vi "Lockin - Format Results.vi"(8 "error in (no error)":errorcluster, 10 "signal in":waveform(dbl)[](array[waveform]), 11 "LockinDAQ":refnum<class "LockinDAQ.lvclass">) -> (0 "error out":errorcluster, 1 "SweepResults":T1, 2 "Results (X,Y,R,Theta)":dbl[][](array[numeric]), 3 "LockinDAQ out":refnum<class "LockinDAQ.lvclass">)   [LabVIEW 2016, in "LockinDAQ.lvclass"]
uses:
  LockinDAQ.lvclass
  Typedefs/SweepResults--Cluster.ctl
  <vilib>/measure/maresamp.llb/Resample Waveform (single shot).vi
  <vilib>/measure/NI_MAPro.lvlib
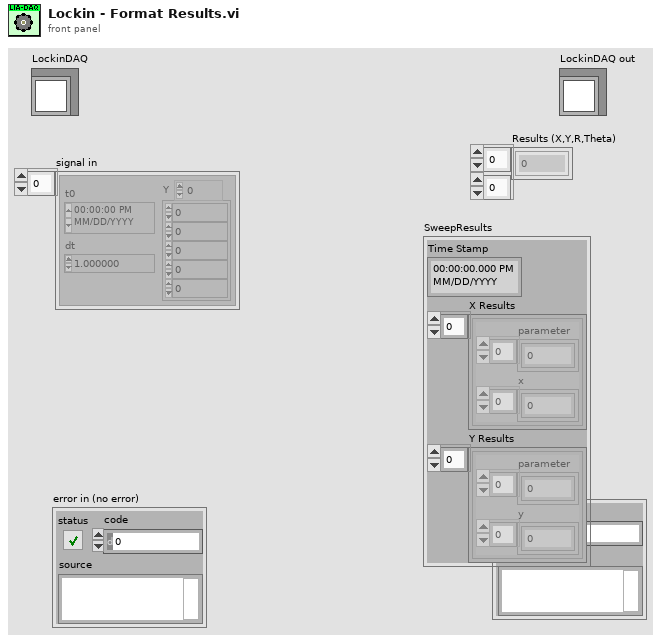
[diagram p1: front panel]
types:
  T1 = typedef "LockinDAQ.lvclass/SweepResults--Cluster.ctl" = cluster{"Time Stamp":timestamp, "X Results":cluster{"parameter":dbl[], "x":dbl[]}[], "Y Results":cluster{"parameter":dbl[], "y":dbl[]}[]}
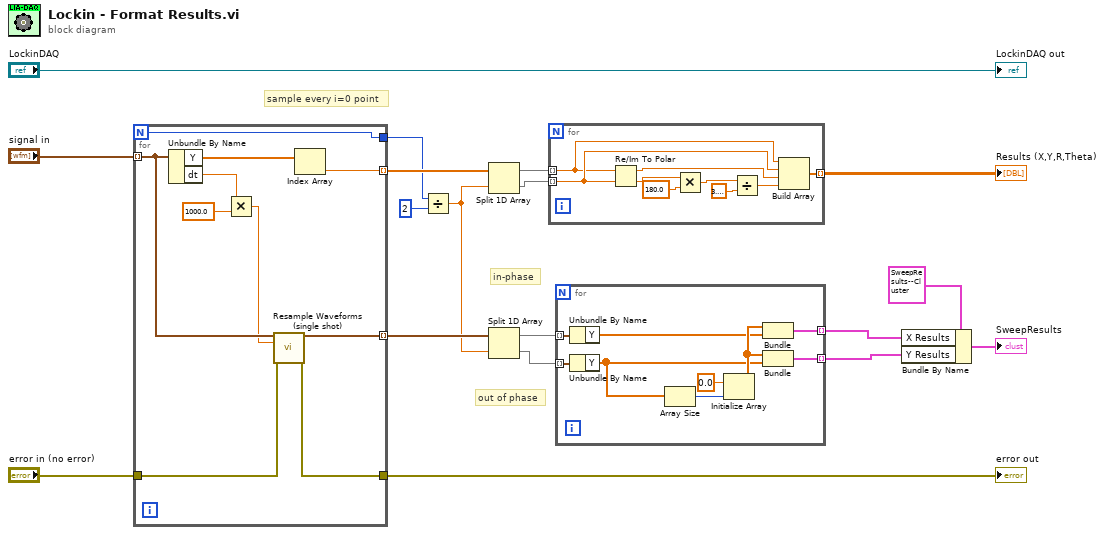
[diagram p0: block diagram]
diagram:
  # "in-phase"
  # "out of phase"
  # "sample every i=0 point"
  n1 = for {
    N -> [w26]
    tunnel: "signal in" -> [w23] mode=indexing
    tunnel: [w28] -> w16 mode=indexing
    tunnel: [w26] -> w15
    tunnel: [w25] -> w13 mode=indexing
    tunnel: "error in (no error)" -> [w20]
    tunnel: [w19] -> w6
    n2 = Unbundle By Name(w23) -> ("Y"=w27:dbl[], "dt"=w22:dbl)
    n3 = Multiply(x=w22, y=1000.0) -> (x*y=w21:dbl)
    n4 = call-poly <vilib>:"Resample Waveforms (single shot).vi"("waveform in"=w23, "dt"=w21, "error in (no error)"=w20) -> ("resampled waveform out"=w25:waveform(dbl), "error out"=w19:errorcluster)  [unwired: 9 in, 2 out]
    n5 = Index Array(array=w27) -> (element=w28:dbl)  [unwired: 1 in]
  }
  "error out" <- w6
  n6 = Divide(x=w15, y=2) -> (x/y=w12:dbl)
  n7 = Split 1D Array(array=w16, index=w12) -> (first subarray=w3:dbl[], second subarray=w1:dbl[])
  n8 = Split 1D Array(array=w13, index=w12) -> (first subarray=w10:waveform(dbl)[], second subarray=w2:waveform(dbl)[])
  n9 = for {
    tunnel: w3 -> [w29] mode=indexing
    tunnel: w1 -> [w31] mode=indexing
    tunnel: [w37] -> w18 mode=indexing
    n10 = Re/Im To Polar(2:w31, 3:w29) -> (0:w35:dbl, 1:w30:dbl)
    n11 = Multiply(x=w35, y=180.0) -> (x*y=w36:dbl)
    n12 = Divide(x=w36, y=3.141592653589793) -> (x/y=w32:dbl)
    n13 = Build Array(w29, w31, w30, w32) -> (w37:dbl[])
  }
  "Results (X,Y,R,Theta)" <- w18
  n14 = for {
    tunnel: w10 -> [w46] mode=indexing
    tunnel: w2 -> [w45] mode=indexing
    tunnel: [w44] -> w5 mode=indexing
    tunnel: [w43] -> w4 mode=indexing
    n15 = Unbundle By Name(w46) -> ("Y"=w39:dbl[])
    n16 = Unbundle By Name(w45) -> ("Y"=w38:dbl[])
    n17 = Array Size(array=w38) -> (size(s)=w41:i32)
    n18 = Initialize Array(0.0 ("element"), w41) -> (w40:dbl[])
    n19 = Bundle(w40, "Y"=w39) -> (w44:cluster{dbl[], "Y":dbl[]})  [unwired: 1 in]
    n20 = Bundle(w40, "Y"=w38) -> (w43:cluster{dbl[], "Y":dbl[]})  [unwired: 1 in]
  }
  n21 = Bundle By Name(cluster=T1 {"Time Stamp"=timestamp(0 s since 1904-01-01), "X Results"=[], "Y Results"=[]} ("SweepResults"), "X Results"=w5, "Y Results"=w4) -> (→"SweepResults":T1)
  "LockinDAQ out" <- "LockinDAQ"
